vi "Webserver_HTML_Download.vi"(7 "password":string="r00t_sola", 9 "IP addres":string="192.168.1.5", 10 "Download path":string="C:\\Temp\\UUT_HMS", 11 "user":string="SolaHD") -> (2 "PASS?":bool)   [LabVIEW 2025]
panel:
  out "cmd output":string
  out "standard error":string
  out "standard output":string
  in  "error in (no error)":errorcluster
  out "error out":errorcluster
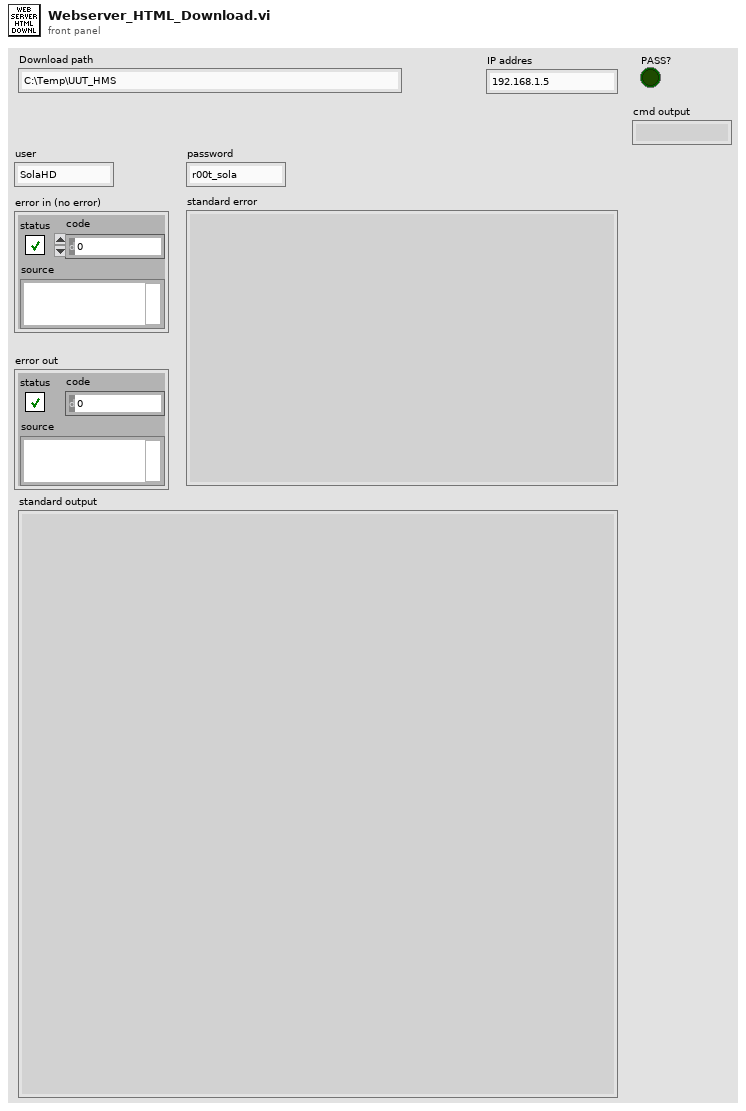
[diagram p1: front panel]
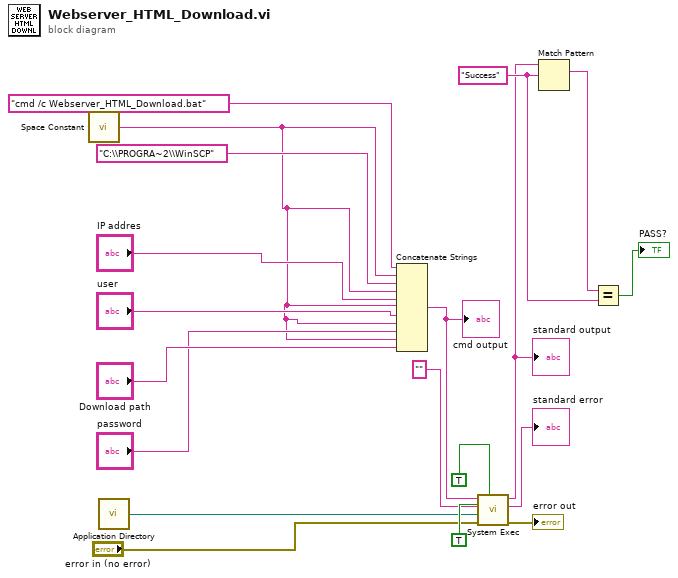
[diagram p0: block diagram]
diagram:
  w10 = "Success" ("text")
  n1 = call <vilib>:"Space Constant.vi"() -> ("String"=w2:string)
  n2 = call <vilib>:"Application Directory.vi"() -> ("Application Directory"=w1:path)
  n3 = Concatenate Strings("cmd /c Webserver_HTML_Download.bat" ("name or relative path"), w2, "C:\\PROGRA~2\\WinSCP" ("WINSCP.exe path"), w2, "IP addres", w2, "user", w2, "password", w2, "Download path") -> (w13:string)
  "cmd output" <- w13
  n4 = call <vilib>:"System Exec.vi"("run minimized? (F)"=TRUE, "wait until completion? (T)"=TRUE ("run minimized? (F)"), "error in (no error)"="error in (no error)", "working directory"=w1, "standard input"="", "command line"=w13) -> ("error out"=→"error out":errorcluster, "standard error"=→"standard error":string, "standard output"=w8:string)  [unwired: 2 in, 1 out]
  "standard output" <- w8
  n5 = Match Pattern(string=w8, regular expression=w10) -> (match substring=w9:string)  [unwired: 1 in, 3 out]
  n6 = Equal?(x=w9, y=w10) -> (x = y?=→"PASS?":bool)
